vi "NUMBER_PAD.vi"() -> (2 "Cancel?":bool, 3 "number (out)":string)   [LabVIEW 2013]
doc: "Modal hexadecimal keypad that allows user to enter a key . If the user presses cancel, the data out is an empty string and the boolean <b>Canceled</b> is set to FALSE."
panel:
  in  "Tab Control":enum32{"Page 1", "Page 2"}(tab)
  in  "F":bool
  in  "E":bool
  in  "D":bool
  in  "C":bool
  in  "B":bool
  in  "A":bool
  in  "Cancel":bool
  in  "Enter":bool
  in  "Clear":bool
  in  "0":bool
  in  "9":bool
  in  "8":bool
  in  "7":bool
  in  "6":bool
  in  "5":bool
  in  "4":bool
  in  "3":bool
  in  "2":bool
  in  "1":bool
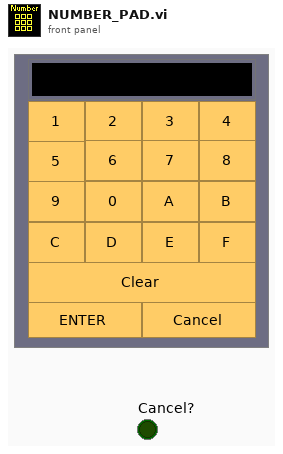
[diagram p1: front panel]
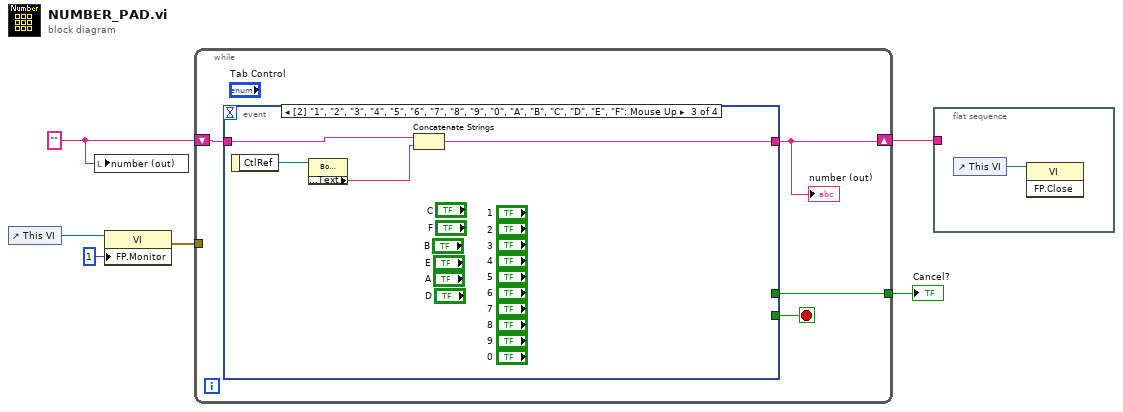
[diagram p0: block diagram]
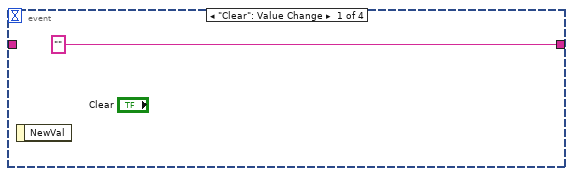
[diagram p2: hidden frame]
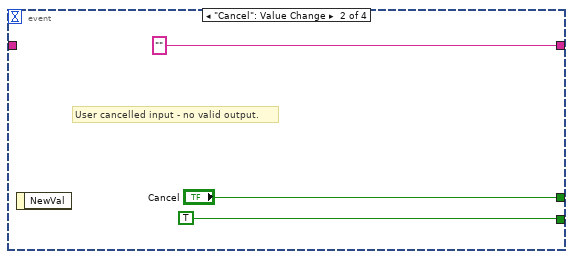
[diagram p3: hidden frame]
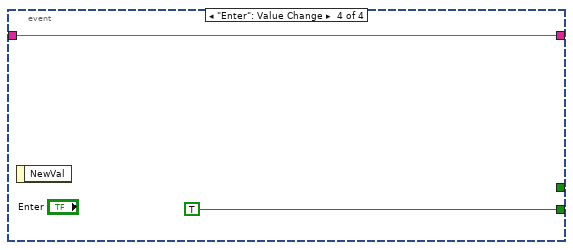
[diagram p4: hidden frame]
diagram:
  w4 = ""
  n1 = control-ref of="This VI"() -> (w3:refnum<vi>)
  n2 = local write "number (out)"(w4) -> ()
  n3 = property class="VI"(reference=w3, "FP.Monitor"=u16 1 ("Front Panel Window:Monitor")) -> (error out=w1:errorcluster)  [unwired: 1 in, 1 out]
  n4 = while {
    shift-right: [w8] -> w6
    shift-left: w4 -> [w10]
    tunnel: [w7] -> w5
    tunnel: w1 -> [_]
    stop <- w9 stop-if-true
    n5 = event shown="[2] \"1\", \"2\", \"3\", \"4\", \"5\", \"6\", \"7\", \"8\", \"9\", \"0\", \"A\", \"B\", \"C\", \"D\", \"E\", \"F\": Mouse Up" {
      selector: _ -> [_ _ _ _]
      dyn-events: _ -> [_ _ _ _]
      timeout: _ -> [_ _ _ _]
      tunnel: w10 -> [_ _ w18 w19]
      tunnel: ["" "" w15 w19] -> w8
      tunnel: [_ TRUE _ TRUE] -> w9
      tunnel: [_ "Cancel" _ _] -> w7
      event "Clear": Value Change {
        n6 = event-data() -> ()  [unwired: 1 in, 1 out]
      }
      event "Cancel": Value Change {
        # "User cancelled input - no valid output."
        n7 = event-data() -> ()  [unwired: 1 in, 1 out]
      }
      event "1", "2", "3", "4", "5", "6", "7", "8", "9", "0", "A", "B", "C", "D", "E", "F": Mouse Up {
        n8 = event-data() -> ("CtlRef"=w17:refnum<vi>)  [unwired: 1 in]
        n9 = property class="Bool (strict)"(reference=w17) -> ("Boolean Text.Text"=w16:string)  [unwired: 1 in, 2 out]
        n10 = Concatenate Strings(w18, w16) -> (w15:string)
      }
      event "Enter": Value Change {
        n11 = event-data() -> ()  [unwired: 1 in, 1 out]
      }
    }
    "number (out)" <- w8
  }
  "Cancel?" <- w5
  n12 = flat-sequence {
    tunnel: w6 -> [_]
    frame #0 {
      n13 = control-ref of="This VI"() -> (w21:refnum<vi>)
      n14 = invoke class="VI" method="FP.Close"(reference=w21) -> ()  [unwired: 2 in, 3 out]
    }
  }
